vi "main_ctrl.vi"(8 "error in":errorcluster) -> (0 "error out":errorcluster caption="error")   [LabVIEW 2013]
uses:
  <vilib>/Rock Robotics/WPI/DriverStation/WPI_DriverStationRobotMode2.ctl
  typedefs/fg_typedef.ctl
  typedefs/vision enable.ctl
  typedefs/vision data.ctl
  typedefs/subStates.ctl
  typedefs/singleUseSubstate.ctl
  <vilib>/Rock Robotics/WPI/Solenoid/WPI_SolenoidValue.ctl
  <vilib>/Rock Robotics/WPI/Compressor/WPI_CompressorGetSetRefNum.vi
  <vilib>/Rock Robotics/WPI/RobotDrive/WPI_RobotDriveGetSetRefNum.vi
  <vilib>/Rock Robotics/WPI/Solenoid/WPI_SolenoidSetEnum.vi
  <vilib>/Rock Robotics/WPI/RobotDrive/WPI_RobotDriveArcadeDrive_Standard(NoSaturation).vi
panel:
  out "Robot Mode":T1
  out "Vision SPI":u32
  out "Vision IPS":dbl
  out "Main IPS":dbl
  out "Main SPI":u32
  # "MAIN CONTROL"
  # "holds robot control code - dual parallel state machine"
  # "SPI: milliseconds per iteration\nIPS: iterations per second"
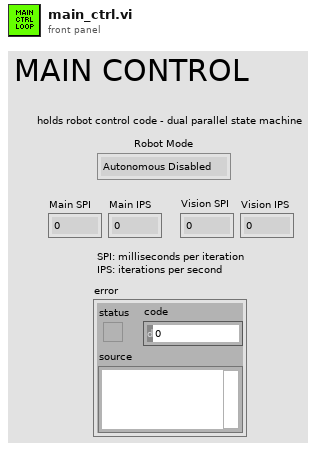
[diagram p1: front panel]
types:
  T1 = typedef "WPI_DriverStationRobotMode2.ctl" = enum16{"Autonomous Disabled", "Autonomous Enabled", "Teleop Disabled", "Teleop Enabled", "Timeout", "Finish", "Test Disabled", "Test Enabled"}
  T2 = typedef "vision data.ctl" = cluster{"x":dbl, "y":dbl, "area":dbl, "width":dbl, "height":dbl, "Hot Goal Present?":bool, "distance":dbl}
  T3 = typedef "vision enable.ctl" = enum16{"Enable", "Disable", "Stop"}
  T4 = typedef "fg_typedef.ctl" = enum16{"Get", "Set"}
  T5 = typedef "WPI_RobotDriveDevRef.ctl" = cluster{"DevStatus":errorcluster, "Motors[]":T6[], "Square Inputs":bool, "Max Output":dbl, "Isochronous":bool}
  T6 = typedef "WPI_MotorControlDeviceRef.ctl" = cluster{"DeviceStatus":errorcluster, "Type":enum16{"PWM", "CAN"}, "PWM":cluster{"Digital Module":T7, "PWM Channel":T8, "DeadBand":T9}, "CAN":cluster{"Device Number":u8, "Control Mode":T10, "Semaphore":T11, "Max Vout":dbl}, "Invert":bool, "TransformRef":T12, "InvTransformRef":T12}
  T7 = typedef "FPGA_TypedefDigitalModule.ctl" = enum16{"Digital Module 1", "Digital Module 2"}
  T8 = typedef "FPGA_DIOPWMChannel.ctl" = enum8{"PWM 1", "PWM 2", "PWM 3", "PWM 4", "PWM 5", "PWM 6", "PWM 7", "PWM 8", "PWM 9", "PWM 10", "Invalid"}
  T9 = typedef "WPI_PWMDeadband.ctl" = cluster{"Name":string, "maxPositivePwm":i32, "minPositivePwm":i32, "centerPwm":i32, "maxNegativePwm":i32, "minNegativePwm":i32, "angularRange":u16}
  T10 = typedef "WPI_CANJaguar_ControlMode.ctl" = enum8{"Percent VBus", "Current", "Speed", "Position", "Voltage"}
  T11 = typedef "Semaphore RefNum" = refnum<k1>
  T12 = typedef "WPI_PWMTransform_ConPane.ctl" = refnum<vi>
  T13 = typedef "WPI_SolenoidDevRef.ctl" = cluster{"DevStatus":errorcluster, "Solenoid Module":T14, "Forward Solenoid Channel":T15, "Reverse Solenoid Channel":T15}
  T14 = typedef "FPGA_TypedefSolenoidModule.ctl" = enum16{"Solenoid Module 1", "Solenoid Module 2"}
  T15 = typedef "WPI_SolenoidChannel.ctl" = enum8{"Solenoid 1", "Solenoid 2", "Solenoid 3", "Solenoid 4", "Solenoid 5", "Solenoid 6", "Solenoid 7", "Solenoid 8", "Invalid"}
  T16 = typedef "WPI_CompressorDevRef.ctl" = cluster{"DevStatus":errorcluster, "DigitalInputDevRef":T17, "RelayDevRef":T19}
  T17 = typedef "WPI_DigitalInputDevRef.ctl" = cluster{"DevStatus":errorcluster, "DIO Channel":T18, "Digital Module":T7}
  T18 = typedef "FPGA_DIOChannel.ctl" = enum8{"DIO 1", "DIO 2", "DIO 3", "DIO 4", "DIO 5", "DIO 6", "DIO 7", "DIO 8", "DIO 9", "DIO 10", "DIO 11", "DIO 12", "DIO 13", "DIO 14", "Invalid"}
  T19 = typedef "WPI_RelayDevRef.ctl" = cluster{"DevStatus":errorcluster, "Relay Channel":T20, "Digital Module":T7, "Relay Direction":T21}
  T20 = typedef "FPGA_DIORelayChannel.ctl" = enum8{"Relay 1", "Relay 2", "Relay 3", "Relay 4", "Relay 5", "Relay 6", "Relay 7", "Relay 8", "Invalid"}
  T21 = typedef "WPI_RelayDirection.ctl" = enum16{"Both directions", "Forward only", "Reverse only"}
  T22 = typedef "WPI_CameraDevRef.ctl" = cluster{"Camera Address":string, "CameraStatus":errorcluster, "Acquire Image Notifier":refnum<notifier>}
  T23 = typedef "IMAQ Image.ctl" = refnum<image>
  T24 = typedef "WPI_SolenoidValue.ctl" = enum16{"Off", "On", "Forward", "Reverse"}
  T25 = typedef "singleUseSubstate.ctl" = enum16{"null", "wait", "shift high", "shift low"}
  T26 = typedef "WPI_DriverStationDerivedRobotMode.ctl" = enum16{"Init", "Execute", "Stop"}
  T27 = typedef "subStates.ctl" = enum16{"null", "wait", "driver control", "auto", "manual override", "hold position", "rotate", "pickup", "pass", "load", "goto shoot", "shoot", "end"}
  T28 = typedef "Loop 2 Datatype.ctl" = cluster{"State":T27, "Waiting Loop":i32, "State to Wait For":i32, "Loop ID":i32, "Exit Value":i32, "Joystick Y":dbl, "Tune Speed":dbl}
  T29 = typedef "Loop 1 Datatype.ctl" = cluster{"State":T27, "Waiting Loop":i32, "State to Wait For":i32, "Loop ID":i32, "Exit Value":i32}
  T30 = typedef "Loop 3 Datatype.ctl" = cluster{"State":T27, "Waiting Loop":i32, "State to Wait For":i32, "Loop ID":i32, "Exit Value":i32, "Joystick Y":dbl, "Joystick Z":dbl}
  T31 = typedef "Loop 0 Datatype.ctl" = cluster{"State":T27, "Waiting Loop":i32, "State to Wait For":i32, "Loop ID":i32, "Exit Value":i32, "X Axis":dbl, "Y Axis":dbl, "Z Axis":dbl}
  T32 = typedef "Loop 4 Datatype.ctl" = cluster{"State":T27, "Waiting Loop":i32, "State to Wait For":i32, "Loop ID":i32, "Exit Value":i32}
  T33 = cluster{"Vision mSPI":u32, "Main mSPI":u32, "Dash mSPI":u32}
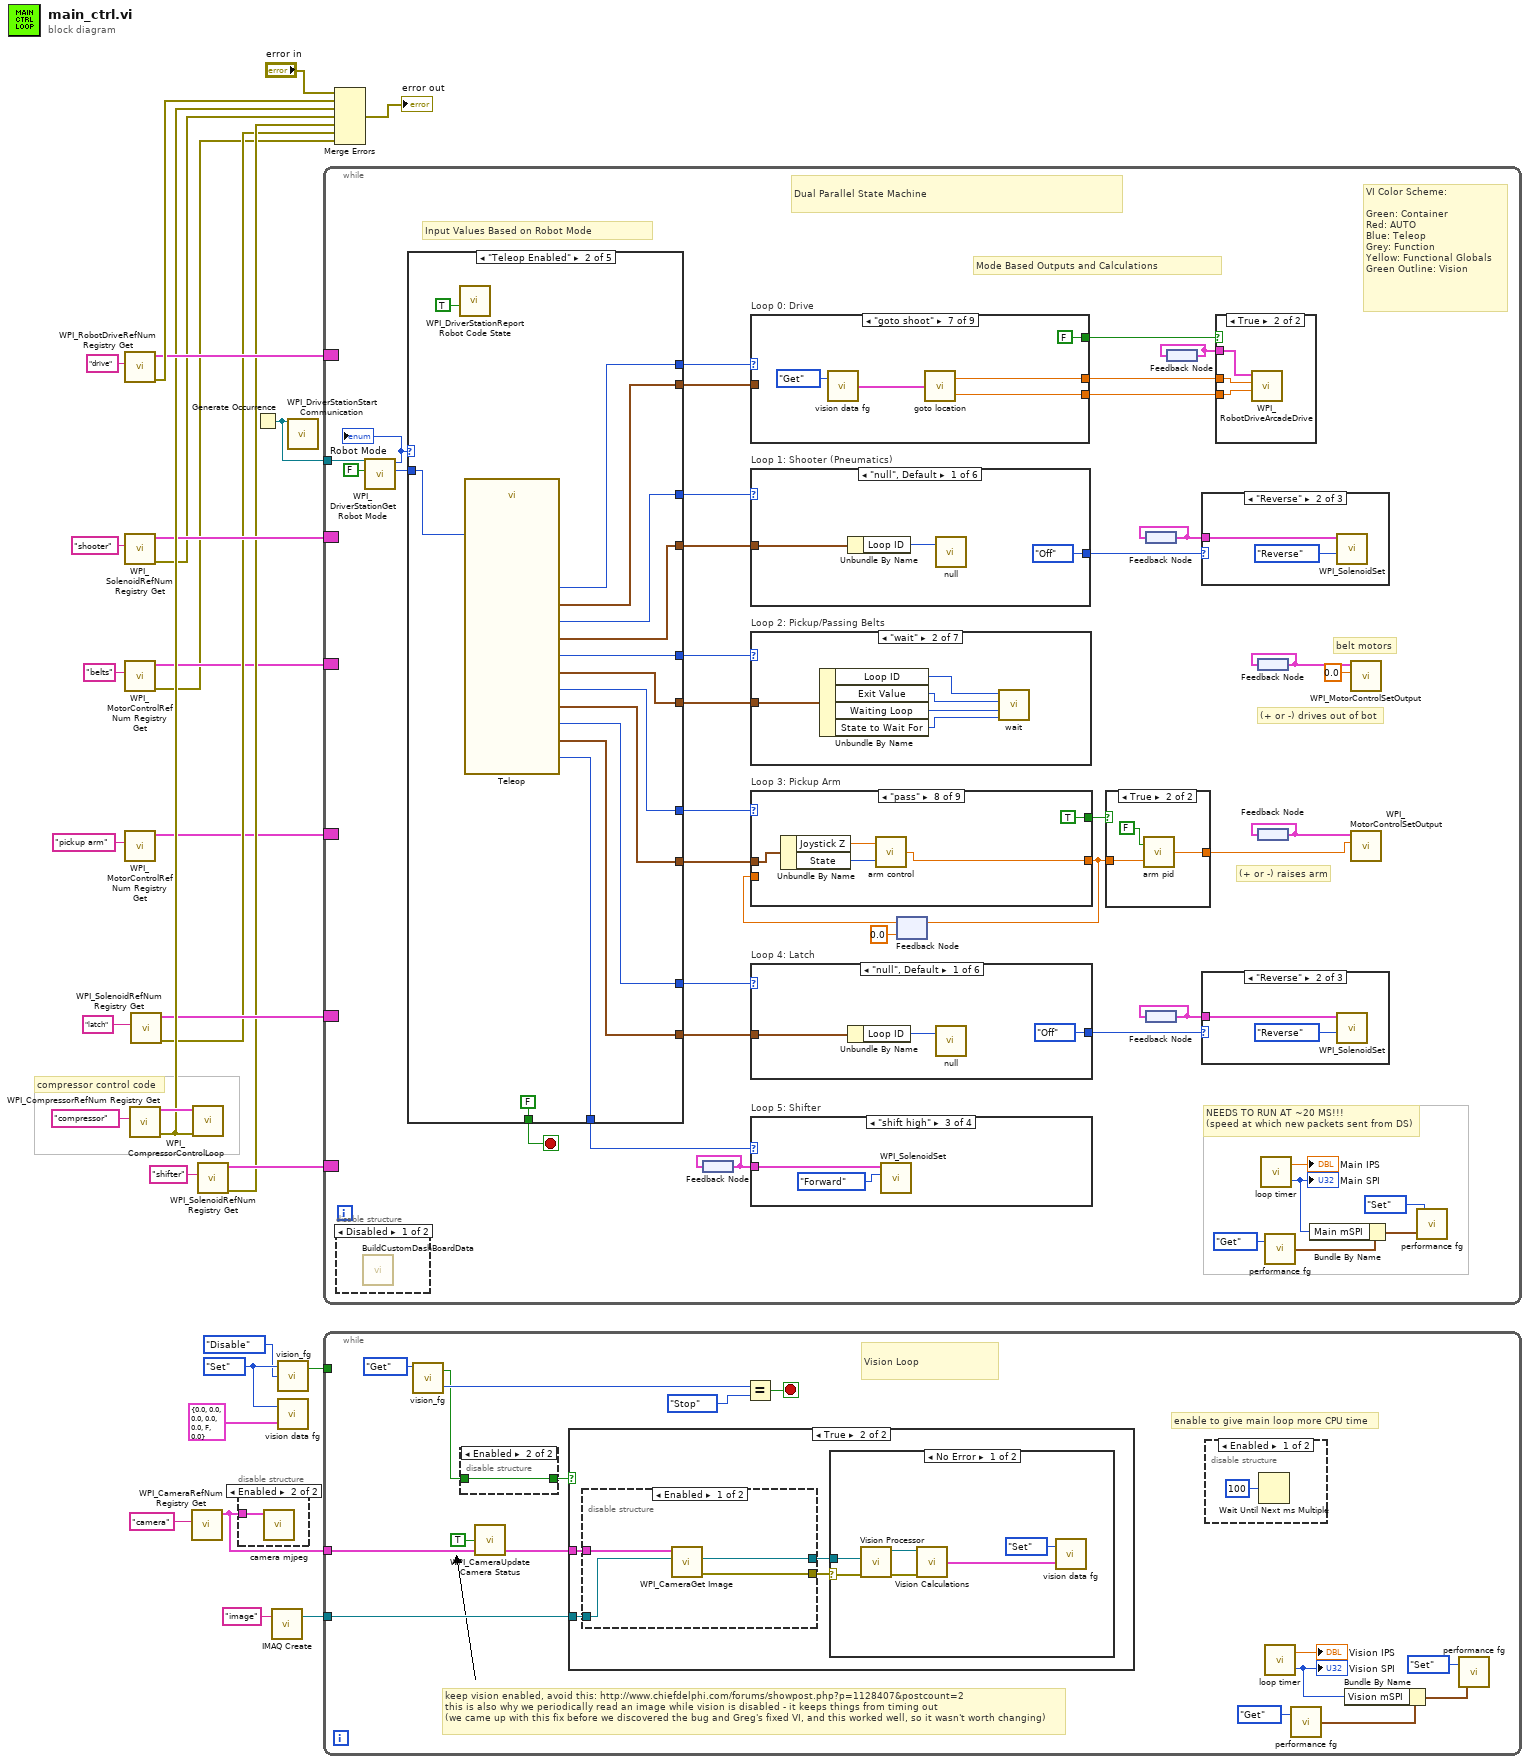
[diagram p0: block diagram]
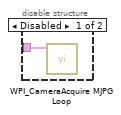
[diagram p2: hidden frame]
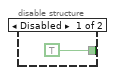
[diagram p3: hidden frame]
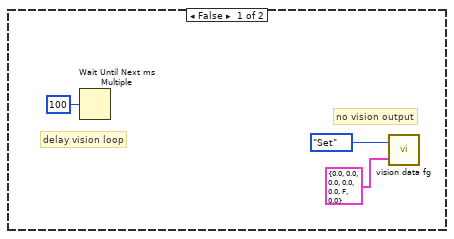
[diagram p5: hidden frame]
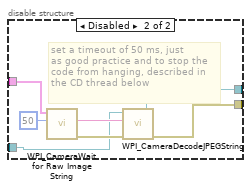
[diagram p7: hidden frame]
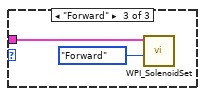
[diagram p10: hidden frame]
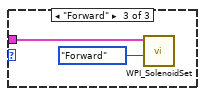
[diagram p12: hidden frame]
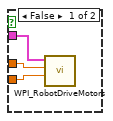
[diagram p14: hidden frame]
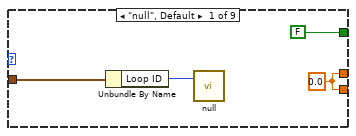
[diagram p15: hidden frame]
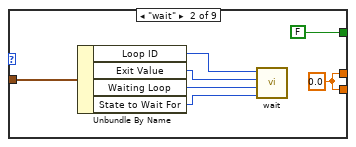
[diagram p16: hidden frame]
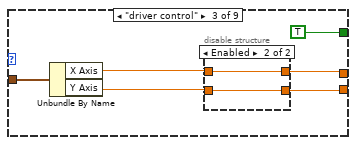
[diagram p17: hidden frame]
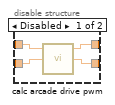
[diagram p18: hidden frame]
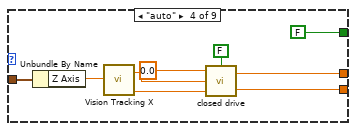
[diagram p19: hidden frame]
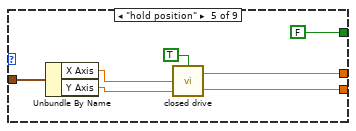
[diagram p20: hidden frame]
diagram:
  w19 = fg_typedef."Set" ("Enum")
  # "compressor control code"
  n1 = call <vilib>:"WPI_RobotDriveRefNum Registry Get.vi"("refnum name"="drive") -> ("error out"=w28:errorcluster, "RobotDriveDevRef"=w26:T5)  [unwired: 9 in]
  n2 = call <vilib>:"WPI_SolenoidRefNum Registry Get.vi"("refnum name"="shooter") -> ("error out"=w7:errorcluster, "SolenoidDevRef"=w11:T13)  [unwired: 9 in]
  n3 = call <vilib>:"WPI_MotorControlRefNum Registry Get.vi"("refnum name"="belts") -> ("error out"=w3:errorcluster, "MotorControlDevRef"=w5:T6)  [unwired: 9 in]
  n4 = call <vilib>:"WPI_MotorControlRefNum Registry Get.vi"("refnum name"="pickup arm") -> ("MotorControlDevRef"=w1:T6)  [unwired: 9 in, 1 out]
  n5 = call <vilib>:"WPI_CompressorRefNum Registry Get.vi"("refnum name"="compressor") -> ("error out"=w22:errorcluster, "CompressorDevRef"=w25:T16)  [unwired: 9 in]
  n6 = call <vilib>:"WPI_SolenoidRefNum Registry Get.vi"("refnum name"="latch") -> ("error out"=w6:errorcluster, "SolenoidDevRef"=w9:T13)  [unwired: 9 in]
  n7 = call <vilib>:"WPI_CameraRefNum Registry Get.vi"("refnum name"="camera") -> ("CameraDevRef"=w16:T22)  [unwired: 9 in, 1 out]
  n8 = call <vilib>:"WPI_CompressorControlLoop.vi"("error in (no error)"=w22, "CompressorDevRef"=w25) -> ()  [unwired: 10 in]
  n9 = call <vilib>:"WPI_SolenoidRefNum Registry Get.vi"("refnum name"="shifter") -> ("error out"=w8:errorcluster, "SolenoidDevRef"=w24:T13)  [unwired: 9 in]
  n10 = disable-structure shown="Enabled" {
    disable-tunnel: w16 -> [w32 w33]
    frame Disabled {
      n11 = call <vilib>:"WPI_CameraAcquire MJPG Loop.vi"("CameraDevRef"=w32) -> ()  [unwired: 11 in]
    }
    frame Enabled {
      n12 = call "camera mjpeg.vi"("CameraDevRef"=w33) -> ()  [unwired: 11 in]
    }
  }
  n13 = Generate Occurrence() -> (w14:refnum<k4>)
  n14 = call "IMAQ Create"("Image Name"="image") -> ("New Image"=w21:T23)  [unwired: 4 in, 1 out]
  n15 = call "vision_fg.vi"("Action"=vision_enable."Disable", "Menu"=w19) -> ("Enabled?"=w20:bool)  [unwired: 1 in, 1 out]
  n16 = call "vision data fg.vi"("Input"=T2 {"x"=0.0, "y"=0.0, "area"=0.0, "width"=0.0, "height"=0.0, "Hot Goal Present?"=FALSE, "distance"=0.0} ("Cluster"), "Menu"=w19) -> ()  [unwired: 1 out]
  n17 = call <vilib>:"WPI_DriverStationStart Communication.vi"("occurrence"=w14) -> ()  [unwired: 11 in]
  n18 = while {
    tunnel: w14 -> [w48]
    border: w26 -> [_]
    border: w24 -> [_]
    border: w11 -> [_]
    border: w9 -> [_]
    border: w5 -> [_]
    border: w1 -> [_]
    stop <- w69 stop-if-true
    # "(+ or -) raises arm"
    # "(+ or -) drives out of bot"
    # "belt motors"
    # "VI Color Scheme:\n\nGreen: Container\nRed: AUTO\nBlue: Teleop\nGrey: Function\nYellow: Functional Globals\nGreen Outline: Vision"
    # "Input Values Based on Robot Mode"
    # "Mode Based Outputs and Calculations"
    # "NEEDS TO RUN AT ~20 MS!!!\n(speed at which new packets sent from DS)"
    # "Dual Parallel State Machine"
    n19 = disable-structure shown="Disabled" {
      frame Disabled {
        n20 = call "BuildCustomDashBoardData.vi"() -> ()  [unwired: 12 in]
      }
      frame Enabled {
      }
    }
    n21 = call <vilib>:"WPI_DriverStationGet Robot Mode.vi"("Finish"=FALSE, "DS Occurrence"=w48) -> ("Call Context"=w47:T26, "Robot Mode"=w46:T1)  [unwired: 8 out]
    "Robot Mode" <- w46
    n22 = case shown="\"Teleop Enabled\"" w46 {
      tunnel: [w239 w256 w258 w264 w270] -> w50
      tunnel: w47 -> [w230 w252 _ _ _]
      tunnel: [w237 w255 w258 w264 w270] -> w71
      tunnel: [w231 w253 singleUseSubstate."null" ("SubState 5") singleUseSubstate."null" ("SubState 5") singleUseSubstate."null" ("SubState 5")] -> w70
      tunnel: [FALSE FALSE FALSE FALSE TRUE] -> w69
      tunnel: [w241 w251 w258 w264 w270] -> w62
      tunnel: [w240 w250 _ _ _] -> w63
      tunnel: [w238 w249 _ _ _] -> w61
      tunnel: [w236 w248 _ _ _] -> w60
      tunnel: [w234 w247 _ _ _] -> w58
      tunnel: [w232 w246 _ _ _] -> w57
      tunnel: [w233 w245 w258 w264 w270] -> w56
      tunnel: [w235 w244 w258 w264 w270] -> w55
      frame "Autonomous Enabled" {
        n23 = call <vilib>:"WPI_DriverStationReport Robot Code State.vi"("Autonomous"=TRUE) -> ()  [unwired: 10 in, 1 out]
        n24 = call "Autonomous.vi"("Call Context"=w230) -> ("SubState 2"=w237:T27, "Loop 2 Data"=w236:T28, "SubState 1"=w239:T27, "Loop 1 Data"=w238:T29, "Loop 3 Data"=w234:T30, "SubState 0"=w241:T27, "SubState 3"=w235:T27, "Loop 0 Data"=w240:T31, "Loop 4 Data"=w232:T32, "SubState 4"=w233:T27, "SubState 5"=w231:T25)
      }
      frame "Teleop Enabled" {
        n25 = call <vilib>:"WPI_DriverStationReport Robot Code State.vi"("TeleOp"=TRUE) -> ()  [unwired: 10 in, 1 out]
        n26 = call "Teleop.vi"("Call Context"=w252) -> ("SubState 3"=w244:T27, "SubState 4"=w245:T27, "SubState 5"=w253:T25, "Loop 3 Data"=w247:T30, "Loop 4 Data"=w246:T32, "SubState 0"=w251:T27, "Loop 1 Data"=w249:T29, "Loop 0 Data"=w250:T31, "SubState 1"=w256:T27, "Loop 2 Data"=w248:T28, "SubState 2"=w255:T27)  [unwired: 8 in]
      }
      frame "Autonomous Disabled", "Teleop Disabled", "Timeout" {
        w258 = subStates."null" ("SubState 0")
        # "set all loops to null"
        # "make sure to disable vision\nwe don't need it here"
        # "robot disabled, timeout"
        n27 = call <vilib>:"WPI_DriverStationReport Robot Code State.vi"("Disabled"=TRUE) -> ()  [unwired: 10 in, 1 out]
        n28 = call "vision_fg.vi"("Action"=vision_enable."Disable", "Menu"=fg_typedef."Set") -> ()  [unwired: 1 in, 2 out]
      }
      frame "Test Disabled", "Test Enabled" {
        w264 = subStates."null" ("SubState 0")
        # "set all loops to null"
        # "make sure to disable vision\nwe don't need it here"
        # "test, unused"
        n29 = call <vilib>:"WPI_DriverStationReport Robot Code State.vi"("Test"=TRUE) -> ()  [unwired: 10 in, 1 out]
        n30 = call "vision_fg.vi"("Action"=vision_enable."Disable", "Menu"=fg_typedef."Set") -> ()  [unwired: 1 in, 2 out]
      }
      frame "Finish" {
        w270 = subStates."end"  # Stop All Loops
        # "stop the while loop"
        # "stop DS comms"
        # "stop vision loop"
        n31 = call <vilib>:"WPI_DriverStationStop Communication.vi"("StopCommunication"=TRUE) -> ()  [unwired: 10 in, 1 out]
        n32 = call "vision_fg.vi"("Action"=vision_enable."Stop", "Menu"=fg_typedef."Set") -> ()  [unwired: 1 in, 2 out]
      }
    }
    n33 = feedback #1() -> (w59:T13)
    n34 = feedback-in #1(w59) -> ()
    n35 = case "Loop 0: Drive" shown="\"goto shoot\"" w62 {
      tunnel: w63 -> [w93 w97 w107 w116 w128 w135 _ _ w151]
      tunnel: [w91 w95 w103 w121 w125 w137 w140 w145 w147] -> w53
      tunnel: [w91 w95 w102 w120 w124 w136 w139 w145 w146] -> w52
      tunnel: [FALSE FALSE TRUE FALSE FALSE FALSE FALSE FALSE FALSE] -> w54
      frame "null", Default {
        w91 = 0.0 ("X Axis")
        n36 = Unbundle By Name(w93) -> ("Loop ID"=w94:i32)
        n37 = call "null.vi"("This Loop ID"=w94) -> ()  [unwired: 2 in]
      }
      frame "wait" {
        w95 = 0.0 ("X Axis")
        n38 = Unbundle By Name(w97) -> ("Loop ID"=w101:i32, "Exit Value"=w100:i32, "Waiting Loop"=w99:i32, "State to Wait For"=w98:i32)
        n39 = call "wait.vi"("State to wait for"=w98, "Waiting Loop ID"=w99, "time (ms)"=w100, "Current Loop ID"=w101) -> ()  [unwired: 1 out]
      }
      frame "driver control" {
        n40 = Unbundle By Name(w107) -> ("X Axis"=w105:dbl, "Y Axis"=w104:dbl)
        n41 = disable-structure shown="Enabled" {
          disable-tunnel: w105 -> [w111 w113]
          disable-tunnel: w104 -> [w110 w112]
          disable-tunnel: [w109 w113] -> w103
          disable-tunnel: [w108 w112] -> w102
          frame Disabled {
            n42 = call "calc arcade drive pwm.vi"("Y axis value"=w110, "X axis value"=w111) -> ("Right Speed"=w108:dbl, "Left Speed"=w109:dbl)  [unwired: 1 in, 1 out]
          }
          frame Enabled {
          }
        }
      }
      frame "auto" {
        n43 = Unbundle By Name(w116) -> ("Z Axis"=w114:dbl)
        n44 = call "Vision Tracking X.vi"("Tweak"=w114) -> ("right speed"=w115:dbl, "left speed"=w118:dbl)
        n45 = call "closed drive.vi"("Acrade Drive?"=FALSE, "Y axis value (Left)"=w118, "X axis value (Right)"=w115, "Threshold (.4)"=0.0 ("Threshold")) -> ("right"=w120:dbl, "left"=w121:dbl)
      }
      frame "hold position" {
        n46 = Unbundle By Name(w128) -> ("X Axis"=w127:dbl, "Y Axis"=w126:dbl)
        n47 = call "closed drive.vi"("Acrade Drive?"=TRUE, "Y axis value (Left)"=w126, "X axis value (Right)"=w127) -> ("right"=w124:dbl, "left"=w125:dbl)  [unwired: 1 in]
      }
      frame "rotate" {
        # "use these to carry actual information because this is\nfor autonomous only so there will not be joystick input"
        n48 = Unbundle By Name(w135) -> ("X Axis"=w134:dbl, "Y Axis"=w133:dbl)
        n49 = call "rotate.vi"("Angle"=w134, "Rate"=w133) -> ("finished?"=w130:bool, "left speed"=w137:dbl, "right speed"=w136:dbl)
        n50 = call "states FG.vi"("exit in"=w130, "menu (get)"=enum16{"set", "get"}."set", "Loop ID"=0) -> ()  [unwired: 5 in, 4 out]
      }
      frame "goto shoot" {
        n51 = call "vision data fg.vi"("Menu"=fg_typedef."Get") -> ("Output"=w141:T2)  [unwired: 1 in]
        n52 = call "goto location.vi"("Image Data"=w141) -> ("left speed"=w140:dbl, "right speed"=w139:dbl)
      }
      frame "end" {
        w145 = 0.0 ("X Axis")
      }
      frame "manual override" {
        n53 = Unbundle By Name(w151) -> ("X Axis"=w150:dbl, "Y Axis"=w149:dbl)
        n54 = expression code="x/2"(w150) -> (w147:dbl)
        n55 = expression code="x/2"(w149) -> (w146:dbl)
      }
    }
    n56 = case "Loop 1: Shooter (Pneumatics)" shown="\"null\", Default" w50 {
      tunnel: w61 -> [w217 w220 _ _ _ _]
      tunnel: [WPI_SolenoidValue."Off" ("Value") WPI_SolenoidValue."Off" ("Value") WPI_SolenoidValue."Off" ("Value") WPI_SolenoidValue."Reverse" ("Value") WPI_SolenoidValue."Off" ("Value") WPI_SolenoidValue."Forward" ("Value")] -> w45
      frame "null", Default {
        n57 = Unbundle By Name(w217) -> ("Loop ID"=w218:i32)
        n58 = call "null.vi"("This Loop ID"=w218) -> ()  [unwired: 2 in]
      }
      frame "wait" {
        n59 = Unbundle By Name(w220) -> ("Loop ID"=w224:i32, "Exit Value"=w223:i32, "Waiting Loop"=w222:i32, "State to Wait For"=w221:i32)
        n60 = call "wait.vi"("State to wait for"=w221, "Waiting Loop ID"=w222, "time (ms)"=w223, "Current Loop ID"=w224) -> ()  [unwired: 1 out]
      }
      frame "driver control" {
      }
      frame "auto" {
        # "retracts cocking pistions"
      }
      frame "manual override" {
      }
      frame "load" {
        # "need actual code instead of this here"
      }
    }
    n61 = case "Loop 2: Pickup/Passing Belts" shown="\"wait\"" w71 {
      tunnel: w60 -> [w210 w211 _ _ _ _ _]
      frame "null", Default {
        n62 = Unbundle By Name(w210) -> ("Loop ID"=w209:i32)
        n63 = call "null.vi"("This Loop ID"=w209) -> ()  [unwired: 2 in]
      }
      frame "wait" {
        n64 = Unbundle By Name(w211) -> ("Loop ID"=w215:i32, "Exit Value"=w214:i32, "Waiting Loop"=w213:i32, "State to Wait For"=w212:i32)
        n65 = call "wait.vi"("State to wait for"=w212, "Waiting Loop ID"=w213, "time (ms)"=w214, "Current Loop ID"=w215) -> ()  [unwired: 1 out]
      }
      frame "driver control" {
      }
      frame "auto" {
      }
      frame "manual override" {
      }
      frame "pickup" {
      }
      frame "load" {
      }
    }
    n66 = case "Loop 4: Latch" shown="\"null\", Default" w56 {
      tunnel: w57 -> [w154 w156 _ _ _ _]
      tunnel: [WPI_SolenoidValue."Off" ("Value") WPI_SolenoidValue."Off" ("Value") WPI_SolenoidValue."Off" ("Value") WPI_SolenoidValue."Reverse" ("Value") WPI_SolenoidValue."Forward" ("Value") WPI_SolenoidValue."Off" ("Value")] -> w42
      frame "null", Default {
        n67 = Unbundle By Name(w154) -> ("Loop ID"=w153:i32)
        n68 = call "null.vi"("This Loop ID"=w153) -> ()  [unwired: 2 in]
      }
      frame "wait" {
        n69 = Unbundle By Name(w156) -> ("Loop ID"=w160:i32, "Exit Value"=w159:i32, "Waiting Loop"=w158:i32, "State to Wait For"=w157:i32)
        n70 = call "wait.vi"("State to wait for"=w157, "Waiting Loop ID"=w158, "time (ms)"=w159, "Current Loop ID"=w160) -> ()  [unwired: 1 out]
      }
      frame "driver control" {
      }
      frame "shoot" {
        # "aka disengage"
      }
      frame "auto" {
        # "aka engage"
      }
      frame "manual override" {
      }
    }
    n71 = case "Loop 5: Shifter" shown="\"shift high\"" w70 {
      tunnel: w59 -> [_ _ w206 w207]
      frame "null", Default {
      }
      frame "wait" {
      }
      frame "shift high" {
        n72 = call-poly <vilib>:"WPI_SolenoidSet.vi"("Value"=WPI_SolenoidValue."Forward", "SolenoidDevRef"=w206) -> ()  [unwired: 8 in, 2 out]
      }
      frame "shift low" {
        n73 = call-poly <vilib>:"WPI_SolenoidSet.vi"("Value"=WPI_SolenoidValue."Reverse", "SolenoidDevRef"=w207) -> ()  [unwired: 8 in, 2 out]
      }
    }
    n74 = feedback #2(0.0 ("output")) -> (w35:dbl)
    n75 = case "Loop 3: Pickup Arm" shown="\"pass\"" w55 {
      tunnel: w58 -> [w168 w171 w177 w182 w187 w192 w196 w202 _]
      tunnel: [FALSE FALSE FALSE TRUE FALSE TRUE TRUE TRUE TRUE] -> w38
      tunnel: [0.0 ("output") 0.0 ("output") w176 w179 w185 w188 w193 w198 w203] -> w36
      tunnel: w35 -> [_ _ _ _ _ _ _ _ w203]
      frame "null", Default {
        n76 = Unbundle By Name(w168) -> ("Loop ID"=w167:i32)
        n77 = call "null.vi"("This Loop ID"=w167) -> ()  [unwired: 2 in]
      }
      frame "wait" {
        n78 = Unbundle By Name(w171) -> ("Loop ID"=w175:i32, "Exit Value"=w174:i32, "Waiting Loop"=w173:i32, "State to Wait For"=w172:i32)
        n79 = call "wait.vi"("State to wait for"=w172, "Waiting Loop ID"=w173, "time (ms)"=w174, "Current Loop ID"=w175) -> ()  [unwired: 1 out]
      }
      frame "driver control" {
        n80 = Unbundle By Name(w177) -> ("Joystick Y"=w176:dbl)
      }
      frame "auto" {
        n81 = Unbundle By Name(w182) -> ("Joystick Z"=w181:dbl, "State"=w180:T27)
        n82 = call "arm control.vi"("Z Axis"=w181, "State"=w180) -> ("output"=w179:dbl)  [unwired: 2 in]
      }
      frame "manual override" {
        n83 = Unbundle By Name(w187) -> ("Joystick Y"=w186:dbl)
        n84 = expression code="x/2"(w186) -> (w185:dbl)
      }
      frame "pickup" {
        n85 = Unbundle By Name(w192) -> ("Joystick Z"=w190:dbl, "State"=w189:T27)
        n86 = call "arm control.vi"("Z Axis"=w190, "State"=w189) -> ("output"=w188:dbl)  [unwired: 2 in]
      }
      frame "load" {
        n87 = Unbundle By Name(w196) -> ("Joystick Z"=w195:dbl, "State"=w194:T27)
        n88 = call "arm control.vi"("Z Axis"=w195, "State"=w194) -> ("output"=w193:dbl)  [unwired: 2 in]
      }
      frame "pass" {
        n89 = Unbundle By Name(w202) -> ("Joystick Z"=w200:dbl, "State"=w199:T27)
        n90 = call "arm control.vi"("Z Axis"=w200, "State"=w199) -> ("output"=w198:dbl)  [unwired: 2 in]
      }
      frame "hold position" {
      }
    }
    n91 = feedback-in #2(w36) -> ()
    n92 = case shown="True" w38 {
      tunnel: w36 -> [w73 w76]
      tunnel: [w73 w75] -> w37
      frame False {
        # "open loop"
      }
      frame True {
        n93 = call "arm pid.vi"("Setpoint"=w76, "Autotune?"=FALSE) -> ("Output"=w75:dbl)
      }
    }
    n94 = feedback #3() -> (w44:T13)
    n95 = feedback-in #3(w44) -> ()
    n96 = feedback #4() -> (w43:T13)
    n97 = feedback-in #4(w43) -> ()
    n98 = feedback #5() -> (w51:T5)
    n99 = feedback-in #5(w51) -> ()
    n100 = case shown="\"Reverse\"" w45 {
      tunnel: w44 -> [_ w81 w83]
      frame "Off", Default {
      }
      frame "Reverse" {
        n101 = call-poly <vilib>:"WPI_SolenoidSet.vi"("Value"=WPI_SolenoidValue."Reverse", "SolenoidDevRef"=w81) -> ()  [unwired: 8 in, 2 out]
      }
      frame "Forward" {
        n102 = call-poly <vilib>:"WPI_SolenoidSet.vi"("Value"=WPI_SolenoidValue."Forward", "SolenoidDevRef"=w83) -> ()  [unwired: 8 in, 2 out]
      }
    }
    n103 = case shown="\"Reverse\"" w42 {
      tunnel: w43 -> [_ w77 w79]
      frame "Off", Default {
      }
      frame "Reverse" {
        n104 = call-poly <vilib>:"WPI_SolenoidSet.vi"("Value"=WPI_SolenoidValue."Reverse", "SolenoidDevRef"=w77) -> ()  [unwired: 8 in, 2 out]
      }
      frame "Forward" {
        n105 = call-poly <vilib>:"WPI_SolenoidSet.vi"("Value"=WPI_SolenoidValue."Forward", "SolenoidDevRef"=w79) -> ()  [unwired: 8 in, 2 out]
      }
    }
    n106 = case shown="True" w54 {
      tunnel: w53 -> [w86 w90]
      tunnel: w52 -> [w85 w89]
      tunnel: w51 -> [w87 w88]
      frame False {
        n107 = call <vilib>:"WPI_RobotDriveMotors.vi"("RightSpeed"=w85, "LeftSpeed"=w86, "RobotDriveDevRef"=w87) -> ()  [unwired: 6 in, 3 out]
      }
      frame True {
        n108 = call-poly <vilib>:"WPI_RobotDriveArcadeDrive.vi"("Y axis value"=w89, "X axis value"=w90, "RobotDriveDevRef"=w88) -> ()  [unwired: 6 in, 3 out]
      }
    }
    n109 = feedback #6() -> (w41:T6)
    n110 = feedback-in #6(w41) -> ()
    n111 = feedback #7() -> (w40:T6)
    n112 = feedback-in #7(w40) -> ()
    n113 = call "loop timer.vi"() -> ("IPS"=→"Main IPS":dbl, "SPI"=w68:u32)  [unwired: 1 in]
    "Main SPI" <- w68
    n114 = call "performance fg.vi"("Menu"=fg_typedef."Get") -> ("Output"=w65:T33)  [unwired: 1 in]
    n115 = Bundle By Name(cluster=w65, "Main mSPI"=w68) -> (w64:T33)
    n116 = call <vilib>:"WPI_MotorControlSetOutput.vi"("Output"=0.0, "MotorControlDevRef"=w41) -> ()  [unwired: 7 in, 3 out]
    n117 = call <vilib>:"WPI_MotorControlSetOutput.vi"("Output"=w37, "MotorControlDevRef"=w40) -> ()  [unwired: 7 in, 3 out]
    n118 = call "performance fg.vi"("Input"=w64, "Menu"=fg_typedef."Set") -> ()  [unwired: 1 out]
  }
  n119 = while {
    tunnel: w21 -> [w289]
    tunnel: w16 -> [w288]
    tunnel: w20 -> [_]
    stop <- w290 stop-if-true
    # "keep vision enabled, avoid this: http://www.chiefdelphi.com/forums/showpost.php?p=1128407&postcount=2\nthis is also why we periodically read an image while vision is disabled - it keeps things from timing out\n(we came up with this fix before we discovered the bug and Greg's fixed VI, and this worked well, so it wasn't worth changing)"
    # "enable to give main loop more CPU time"
    # "Vision Loop"
    n120 = call "vision_fg.vi"("Menu"=fg_typedef."Get" ("Enum")) -> ("State Out"=w284:T3, "Enabled?"=w275:bool)  [unwired: 2 in]
    n121 = disable-structure shown="Enabled" {
      disable-tunnel: [TRUE w292] -> w276
      disable-tunnel: w275 -> [_ w292]
      frame Disabled {
      }
      frame Enabled {
      }
    }
    n122 = call <vilib>:"WPI_CameraUpdate Camera Status.vi"("CameraDevRef In"=w288, "Enable Vision"=TRUE) -> ("CameraDevRef Out"=w287:T22)  [unwired: 3 in]
    n123 = case shown="True" w276 {
      tunnel: w289 -> [_ w300]
      tunnel: w287 -> [_ w299]
      frame False {
        # "no vision output"
        # "delay vision loop"
        n124 = Wait Until Next ms Multiple(millisecond multiple=u32 100) -> ()  [unwired: 1 out]
        n125 = call "vision data fg.vi"("Input"=T2 {"x"=0.0, "y"=0.0, "area"=0.0, "width"=0.0, "height"=0.0, "Hot Goal Present?"=FALSE, "distance"=0.0} ("Cluster"), "Menu"=fg_typedef."Set" ("Enum")) -> ()  [unwired: 1 out]
      }
      frame True {
        n126 = disable-structure shown="Enabled" {
          disable-tunnel: w300 -> [w309 w313]
          disable-tunnel: w299 -> [w310 w315]
          disable-tunnel: [w308 w312] -> w298
          disable-tunnel: [w307 w311] -> w297
          frame Enabled {
            n127 = call <vilib>:"WPI_CameraGet Image.vi"("Image"=w309, "CameraDevRef"=w310) -> ("error out"=w307:errorcluster, "Image Out"=w308:T23)  [unwired: 7 in, 1 out]
          }
          frame Disabled {
            # "set a timeout of 50 ms, just\nas good practice and to stop the \ncode from hanging, described in \nthe CD thread below"
            n128 = call <vilib>:"WPI_CameraWait for Raw Image String.vi"("Timeout in ms (-1)"=50, "CameraDevRef"=w315) -> ("error out"=w317:errorcluster, "String"=w316:string)  [unwired: 3 in, 5 out]
            n129 = call <vilib>:"WPI_CameraDecodeJPEGString.vi"("error in"=w317, "Compressed Image"=w316, "Image In"=w313) -> ("error out"=w311:errorcluster, "Image Out"=w312:T23)  [unwired: 3 out]
          }
        }
        n130 = case shown="No Error" w297 {
          selector: w297 -> [w305 _]
          tunnel: w298 -> [w304 _]
          frame No Error {
            n131 = call "Vision Processor.vi"("error in"=w305, "Image In"=w304) -> ("error out"=w302:errorcluster, "Image Out"=w303:T23)  [unwired: 5 in]
            n132 = call "Vision Calculations.vi"("Image In"=w303, "error in"=w302) -> ("Vision Data"=w301:T2)  [unwired: 3 in]
            n133 = call "vision data fg.vi"("Input"=w301, "Menu"=fg_typedef."Set" ("Enum")) -> ()  [unwired: 1 out]
          }
          frame Error {
          }
        }
      }
    }
    n134 = Equal?(x=w284, y=vision_enable."Stop") -> (x = y?=w290:bool)
    n135 = disable-structure shown="Enabled" {
      frame Enabled {
        n136 = Wait Until Next ms Multiple(millisecond multiple=u32 100) -> ()  [unwired: 1 out]
      }
      frame Disabled {
      }
    }
    n137 = call "loop timer.vi"() -> ("IPS"=→"Vision IPS":dbl, "SPI"=w282:u32)  [unwired: 1 in]
    "Vision SPI" <- w282
    n138 = call "performance fg.vi"("Menu"=fg_typedef."Get") -> ("Output"=w280:T33)  [unwired: 1 in]
    n139 = Bundle By Name(cluster=w280, "Vision mSPI"=w282) -> (w279:T33)
    n140 = call "performance fg.vi"("Input"=w279, "Menu"=fg_typedef."Set") -> ()  [unwired: 1 out]
  }
  n141 = Merge Errors("error in", w28, w22, w7, w8, w6, w3) -> (→"error out":errorcluster)
